vi "SetArmSource.vi"(8 "Error In":errorcluster, 10 "Arm Source":T1, 11 "Keithley 6482 In":refnum<visa-resource-name>) -> (0 "Error Out":errorcluster, 3 "Keithley 6482 Out":refnum<visa-resource-name>)   [LabVIEW 2009, in "Keithley-6482-Visa.lvlib"]
uses:
  <instrlib>/Keithley-6482-Visa9.0/Keithley-6482-Visa.lvlib
  <instrlib>/Keithley-6482-Visa9.0/Public/Controls/ArmSource.ctl
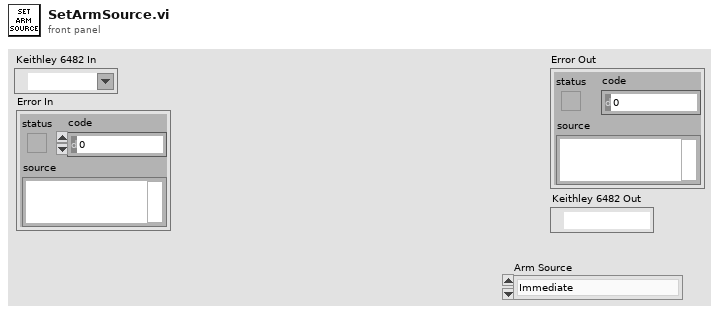
[diagram p1: front panel]
types:
  T1 = typedef "Keithley-6482-Visa.lvlib/ArmSource.ctl" = enum16{"Immediate", "Timer", "Manual", "Bus", "TLink", "NSTest", "PSTest", "BSTest"}
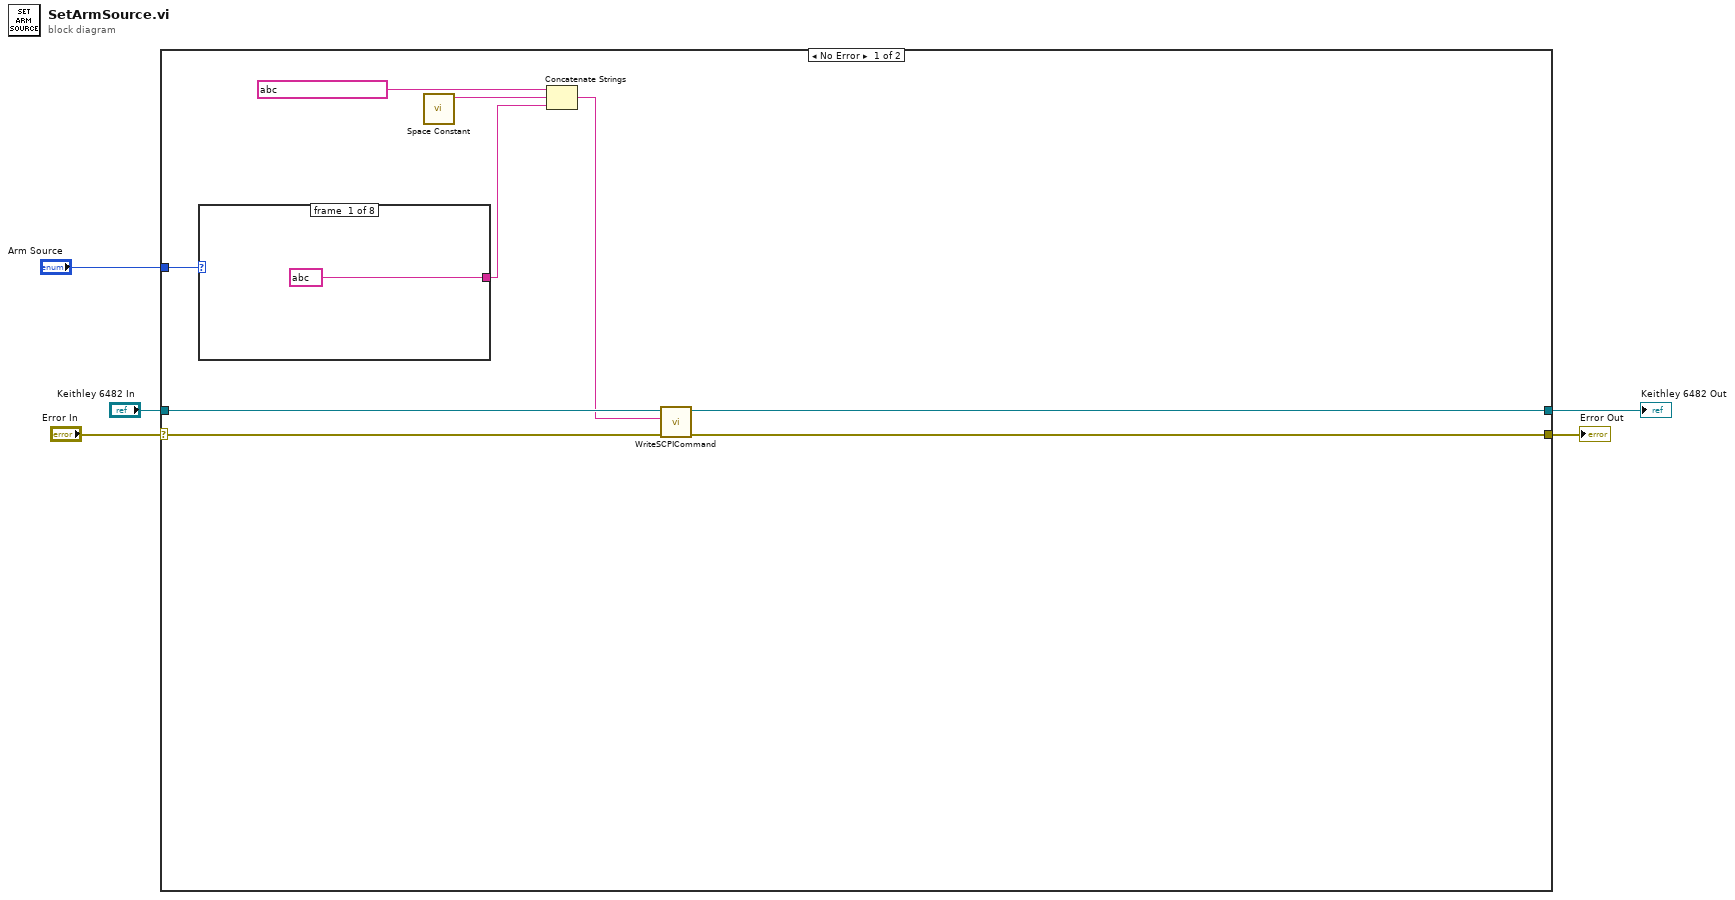
[diagram p0: block diagram]
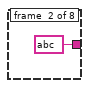
[diagram p2: hidden frame]
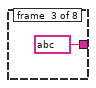
[diagram p3: hidden frame]
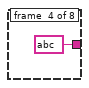
[diagram p4: hidden frame]
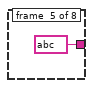
[diagram p5: hidden frame]
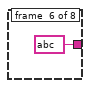
[diagram p6: hidden frame]
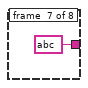
[diagram p7: hidden frame]
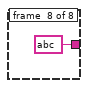
[diagram p8: hidden frame]
diagram:
  n1 = case shown="No Error" "Error In" {
    selector: "Error In" -> [w14 w23]
    tunnel: "Keithley 6482 In" -> [w13 w24]
    tunnel: [w8 w23] -> w3
    tunnel: [w9 w24] -> w2
    tunnel: "Arm Source" -> [w7 _]
    frame #0 {
      n2 = case shown="\"BSTest\"" w7 {
        tunnel: [string ? string ? string ? string ? string ? string ? string ? string ?] -> w6
        frame #0 {
        }
        frame #1 {
        }
        frame #2 {
        }
        frame #3 {
        }
        frame #4 {
        }
        frame #5 {
        }
        frame #6 {
        }
        frame #7 {
        }
      }
      n3 = call <vilib>:"Space Constant.vi"() -> ("String"=w11:string)
      n4 = Concatenate Strings(string ? ("string"), w11, w6) -> (w10:string)
      n5 = call <instrlib>:"WriteSCPICommand.vi"("Error In"=w14, "SCPI Command"=w10, "Keithley 6482 In"=w13) -> ("Error Out"=w8:errorcluster, "Keithley 6482 Out"=w9:refnum<visa-resource-name>)  [unwired: 7 in]
    }
    frame #1 {
    }
  }
  "Error Out" <- w3
  "Keithley 6482 Out" <- w2
